vi "Oscillogram_plugin.vi"() -> (11 "Graph":dynamicdata(graph)=[{"t0"=timestamp(1 s since 1904-01-01), "dt"=1.0, "Y"=array[9999 elements], "attributes"=variant("NI_ChannelName"=variant(string "Voltage (Extracted)"), "NI_ExpIsRelativeTime"=variant(bool TRUE), "NI_ExpStartTimeStamp"=variant(timestamp timestamp(3710244565.071289 s since 1904-01-01)), "NI_ExpTimeStamp"=variant(timestamp timestamp(1 s since 1904-01-01)), "NI_ExpXDimension"=variant(string "t"), "NI_OriginalChannelName"=variant(string "Voltage"))}, {"t0"=timestamp(26 s since 1904-01-01), "dt"=1.0, "Y"=array[9974 elements], "attributes"=variant("NI_ChannelName"=variant(string "Current (Extracted)"), "NI_ExpIsRelativeTime"=variant(bool TRUE), "NI_ExpStartTimeStamp"=variant(timestamp timestamp(3710244565.071289 s since 1904-01-01)), "NI_ExpTimeStamp"=variant(timestamp timestamp(26 s since 1904-01-01)), "NI_ExpXDimension"=variant(string "t"), "NI_OriginalChannelName"=variant(string "Current"))}])   [LabVIEW 2012]
panel:
  in  "Plot":bool=TRUE
  in  "Grid":bool=TRUE
  in  "Main Graph":dynamicdata(graph)=[{"t0"=timestamp(0 s since 1904-01-01), "dt"=1.0, "Y"=array[10000 elements], "attributes"=variant("NI_ChannelName"=variant(string "Voltage"), "NI_ExpIsRelativeTime"=variant(bool TRUE), "NI_ExpStartTimeStamp"=variant(timestamp timestamp(3710244565.071289 s since 1904-01-01)), "NI_ExpTimeStamp"=variant(timestamp timestamp(0 s since 1904-01-01)), "NI_ExpXDimension"=variant(string "t"))}, {"t0"=timestamp(0 s since 1904-01-01), "dt"=1.0, "Y"=array[10000 elements], "attributes"=variant("NI_ChannelName"=variant(string "Current"), "NI_ExpIsRelativeTime"=variant(bool TRUE), "NI_ExpStartTimeStamp"=variant(timestamp timestamp(3710244565.071289 s since 1904-01-01)), "NI_ExpTimeStamp"=variant(timestamp timestamp(0 s since 1904-01-01)), "NI_ExpXDimension"=variant(string "t"))}]
  in  "Line weight":u8=1
  in  "Cursor Color":u32(colorbox)=16711680
  in  "Graph Color":u32(colorbox)=16860
  in  "A Cursor":bool=TRUE
  in  "V Cursor":bool=TRUE
  in  "Y Scale":bool=TRUE
  in  "X Scale":bool=TRUE
  in  "FPS":u32=20000
  in  "Frame counter":u32=10
  out "Current":dbl caption="Current (A)" format="%#.2g"
  out "Voltage":dbl caption="Voltage (V)" format="%#.1f"
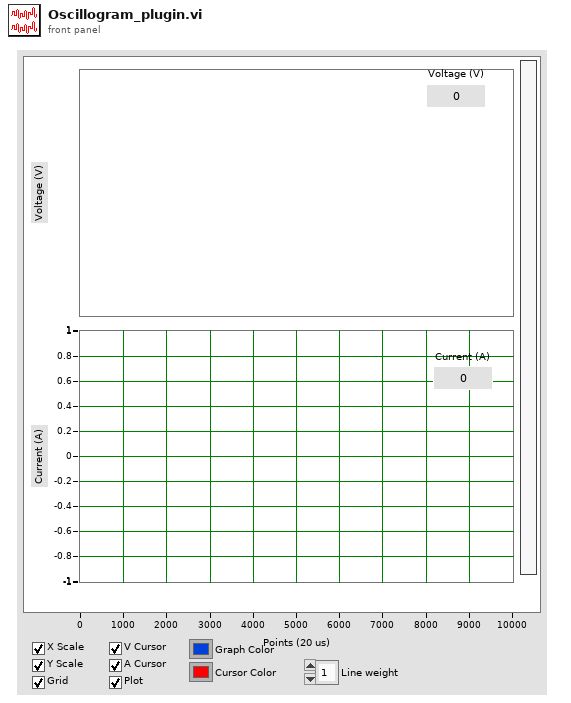
[diagram p1: front panel]
types:
  T1 = typedef "Video_analizer_settings.ctl" = cluster{"Current_shift":dbl, "Video_shift":dbl, "CurrentY_offset":dbl, "VoltageY_offset":dbl, "FIR_enable":bool, "Cutof_freq":dbl, "Order":u32}
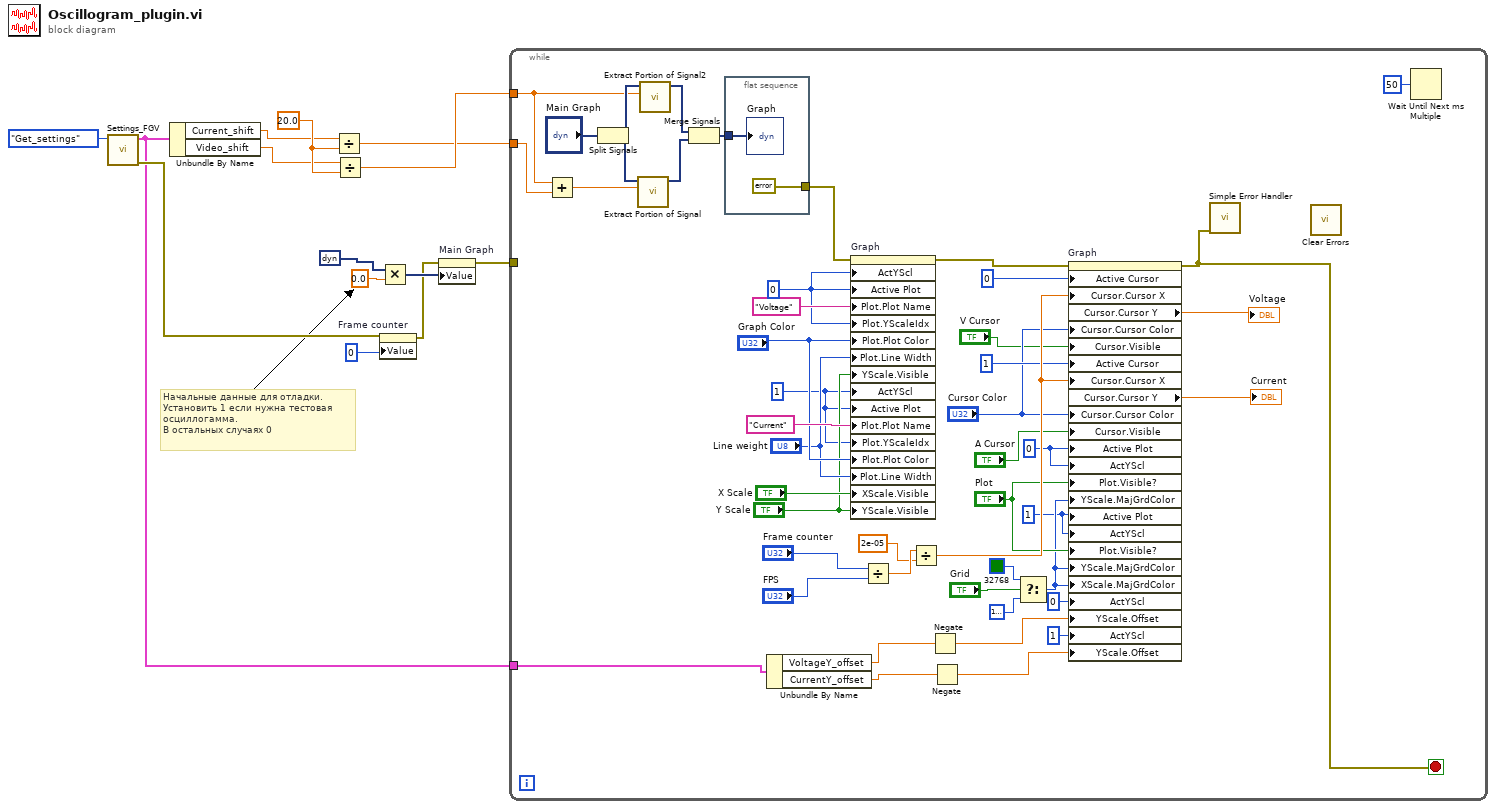
[diagram p0: block diagram]
diagram:
  w7 = 20.0 ("y")
  # "Начальные данные для отладки. \nУстановить 1 если нужна тестовая \nосциллогамма.\nВ остальных случаях 0"
  n1 = call "Settings_FGV.vi"("State"=enum16{"Get_settings", "Set_settings"}."Get_settings") -> ("error out"=w2:errorcluster, "Settings"=w1:T1)  [unwired: 9 in]
  n2 = Unbundle By Name(w1) -> ("Current_shift"=w3:dbl, "Video_shift"=w4:dbl)
  n3 = Divide(x=w3, y=w7) -> (x/y=w5:dbl)
  n4 = Divide(x=w4, y=w7) -> (x/y=w6:dbl)
  n5 = Multiply(x=dynamicdata [{"t0"=timestamp(0 s since 1904-01-01), "dt"=1.0, "Y"=array[10000 elements], "attributes"=variant("NI_ChannelName"=variant(string "Voltage"), "NI_ExpIsRelativeTime"=variant(bool TRUE), "NI_ExpStartTimeStamp"=variant(timestamp timestamp(3710244565.071289 s since 1904-01-01)), "NI_ExpTimeStamp"=variant(timestamp timestamp(0 s since 1904-01-01)), "NI_ExpXDimension"=variant(string "t"))}, {"t0"=timestamp(0 s since 1904-01-01), "dt"=1.0, "Y"=array[10000 elements], "attributes"=variant("NI_ChannelName"=variant(string "Current"), "NI_ExpIsRelativeTime"=variant(bool TRUE), "NI_ExpStartTimeStamp"=variant(timestamp timestamp(3710244565.071289 s since 1904-01-01)), "NI_ExpTimeStamp"=variant(timestamp timestamp(0 s since 1904-01-01)), "NI_ExpXDimension"=variant(string "t"))}] ("Main Graph 2"), y=0.0) -> (x*y=w11:dynamicdata)
  n6 = property on="Frame counter" class="DigNum (strict)"(error in=w2, "Value"=0 ("Frame counter")) -> (error out=w10:errorcluster)  [unwired: 1 in, 1 out]
  n7 = property on="Main Graph" class="MixedGraph (strict)"(error in=w10, "Value"=w11) -> (error out=w14:errorcluster)  [unwired: 1 in, 1 out]
  n8 = while {
    tunnel: w14 -> [_]
    tunnel: w6 -> [w17]
    tunnel: w5 -> [w16]
    tunnel: w1 -> [w20]
    stop <- w49 stop-if-true
    w19 = u32 1 ("Active Plot")
    w18 = u32 0 ("Active Plot")
    w40 = u32 1 ("Active Plot")
    w41 = u32 0 ("Active Plot")
    n9 = Add(x=w17, y=w16) -> (x+y=w28:dbl)
    n10 = Split Signals("Main Graph") -> (w30:dynamicdata, w33:dynamicdata)  [unwired: 2 in]
    n11 = call "Extract Portion of Signal"("Begin Sample"=w28, "Signals"=w33) -> ("Section"=w32:dynamicdata)  [unwired: 8 in, 1 out]
    n12 = call "Extract Portion of Signal2"("Begin Sample"=w17, "Signals"=w30) -> ("Section"=w29:dynamicdata)  [unwired: 8 in, 1 out]
    n13 = Merge Signals(w29, w32) -> (w31:dynamicdata)
    n14 = flat-sequence {
      tunnel: w31 -> [w63]
      tunnel: [errorcluster {"status"=FALSE, "code"=0, "source"=""} ("error out")] -> w15
      frame #0 {
        "Graph" <- w63
      }
    }
    n15 = Unbundle By Name(w20) -> ("VoltageY_offset"=w24:dbl, "CurrentY_offset"=w25:dbl)
    n16 = property on="Graph" class="MixedGraph (strict)"(error in=w15, "ActYScl"=w41, "Active Plot"=w41, "Plot.Plot Name"="Voltage", "Plot.YScaleIdx"=w41, "Plot.Plot Color"="Graph Color", "Plot.Line Width"="Line weight", "YScale.Visible"="Y Scale", "ActYScl"=w40, "Active Plot"=w40, "Plot.Plot Name"="Current", "Plot.YScaleIdx"=w40, "Plot.Plot Color"="Graph Color", "Plot.Line Width"="Line weight", "XScale.Visible"="X Scale", "YScale.Visible"="Y Scale") -> (error out=w50:errorcluster)  [unwired: 1 in, 1 out]
    n17 = Divide(x="Frame counter", y="FPS") -> (x/y=w58:dbl)
    n18 = Divide(x=w58, y=2e-05) -> (x/y=w55:dbl)
    n19 = Negate(x=w24) -> (-x=w23:dbl)
    n20 = Negate(x=w25) -> (-x=w22:dbl)
    n21 = Select(t=u32 32768, s="Grid", f=u32 16777216) -> (s? t:f=w35:u32)
    n22 = property on="Graph" class="MixedGraph (strict)"(error in=w50, "Active Cursor"=u32 0, "Cursor.Cursor X"=w55, "Cursor.Cursor Color"="Cursor Color", "Cursor.Visible"="V Cursor", "Active Cursor"=u32 1, "Cursor.Cursor X"=w55, "Cursor.Cursor Color"="Cursor Color", "Cursor.Visible"="A Cursor", "Active Plot"=w18, "ActYScl"=w18, "Plot.Visible?"="Plot", "YScale.MajGrdColor"=w35, "Active Plot"=w19, "ActYScl"=w19, "Plot.Visible?"="Plot", "YScale.MajGrdColor"=w35, "XScale.MajGrdColor"=w35, "ActYScl"=0 ("Active Y Scale"), "YScale.Offset"=w23, "ActYScl"=1 ("Active Y Scale"), "YScale.Offset"=w22) -> (error out=w49:errorcluster, "Cursor.Cursor Y"=→"Voltage":dbl, "Cursor.Cursor Y"=→"Current":dbl)  [unwired: 1 in, 1 out]
    n23 = call <vilib>:"Simple Error Handler.vi"("error in (no error)"=w49) -> ()  [unwired: 4 in, 5 out]
    n24 = call <vilib>:"Clear Errors.vi"() -> ()  [unwired: 7 in, 1 out]
    n25 = Wait Until Next ms Multiple(millisecond multiple=u32 50) -> ()  [unwired: 1 out]
  }
